vi "Sign.vi"(5 "RSASignPadding":T2, 7 "HashingAlgorithm":T1=enum."SHA512", 8 "error in (no error)":errorcluster, 10 "Data in":u8[](array[numeric]), 11 "CngKey in":refnum<k24>) -> (0 "error out":errorcluster, 2 "Signature out":u8[](array[numeric]), 3 "CngKey out":refnum<k24>)   [LabVIEW 2021, in "dotNET Crypto Asymmetric Encryption.lvlib"]
doc: "Generate a signature from the data using the private key."
uses:
  dotNET Crypto Asymmetric Encryption.lvlib
  RSASignaturePadding.ctl
  HashingAlgorithm.ctl
  System.Core
  Utility/dotNET Crypto Utility.lvlib
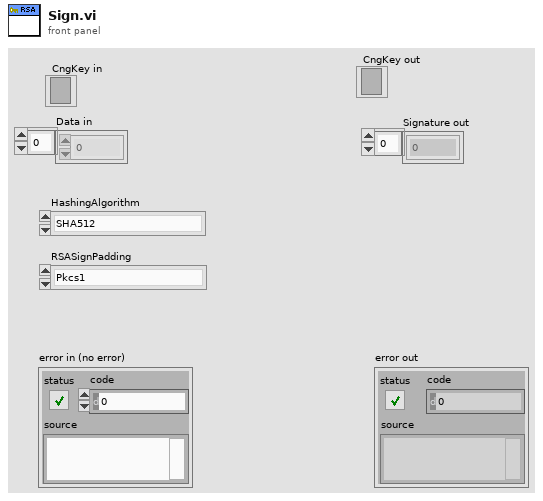
[diagram p1: front panel]
types:
  T1 = typedef "dotNET Crypto Utility.lvlib/HashingAlgorithm.ctl" = enum16{"MD5", "SHA1", "SHA256", "SHA384", "SHA512"}
  T2 = typedef "dotNET Crypto Asymmetric Encryption.lvlib/RSASignaturePadding.ctl" = enum16{"Pkcs1", "Pss"}
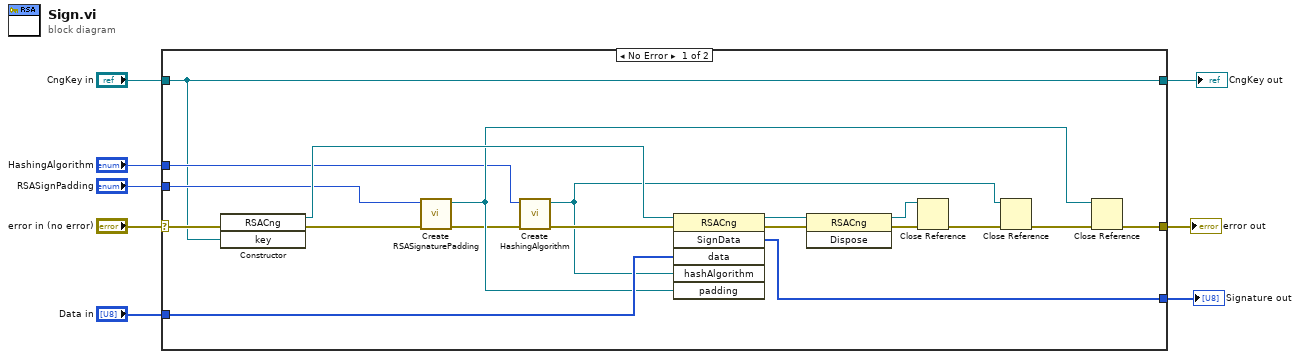
[diagram p0: block diagram]
diagram:
  n1 = case shown="No Error" "error in (no error)" {
    selector: "error in (no error)" -> [w10 w28]
    tunnel: "Data in" -> [w27 _]
    tunnel: [w26 _] -> w7
    tunnel: "RSASignPadding" -> [w18 _]
    tunnel: "HashingAlgorithm" -> [w12 _]
    tunnel: [w11 w28] -> w4
    tunnel: "CngKey in" -> [w9 w29]
    tunnel: [w9 w29] -> w1
    frame No Error {
      n2 = constructor class="RSACng"(error in=w10, "key"=w9) -> (reference out=w20:refnum<k24>, error out=w21:errorcluster)  [unwired: 2 in, 2 out]
      n3 = call "Create RSASignaturePadding.vi"("error in (no error)"=w21, "RSASignaturePadding"=w18) -> ("error out"=w17:errorcluster, "RSASignaturePadding out"=w19:refnum<k24>)  [unwired: 8 in]
      n4 = call "Create HashingAlgorithm.vi"("error in (no error)"=w17, "HashingAlgorithm"=w12) -> ("error out"=w16:errorcluster, "Hashing Algorithm"=w13:refnum<k24>)  [unwired: 8 in]
      n5 = invoke class="RSACng" method="SignData"(reference=w20, error in=w16, "data"=w27, "hashAlgorithm"=w13, "padding"=w19) -> (reference out=w24:refnum<k24>, error out=w25:errorcluster, "SignData"=w26:u8[])  [unwired: 1 in, 3 out]
      n6 = invoke class="RSACng" method="Dispose"(reference=w24, error in=w25) -> (reference out=w23:refnum<k24>, error out=w22:errorcluster)  [unwired: 1 in, 1 out]
      n7 = Close Reference(reference=w23, error in (no error)=w22) -> (error out=w15:errorcluster)
      n8 = Close Reference(reference=w13, error in (no error)=w15) -> (error out=w14:errorcluster)
      n9 = Close Reference(reference=w19, error in (no error)=w14) -> (error out=w11:errorcluster)
    }
    frame Error {
    }
  }
  "error out" <- w4
  "Signature out" <- w7
  "CngKey out" <- w1
